vi "DEMO_08_PID_Use.vi"() -> ()   [LabVIEW 2014]
uses:
  <vilib>/Instr/_visa.llb/VISA Configure Serial Port (Instr).vi
panel:
  in  "停止 3":bool
  in  "停止 2":bool
  in  "停止":bool
  in  "开启 3":bool
  in  "开启 2":bool
  in  "开启":bool
  in  "读取 3":bool
  in  "读取 2":bool
  in  "读取":bool
  in  "P 3":dbl
  in  "设置 3":bool
  in  "D 3":dbl
  in  "I 3":dbl
  in  "P 2":dbl
  in  "设置 2":bool
  in  "D 2":dbl
  in  "I 2":dbl
  in  "P":dbl
  in  "设置":bool
  in  "D":dbl
  in  "I":dbl
  in  "打开串口":bool
  in  "上位机控制":bool
  in  "波特率":u32(ring)=9600 items=["75"=75, "110"=110, "134"=134, "150"=150, "300"=300, "600"=600, "1200"=1200, "1800"=1800, "2400"=2400, "4800"=4800, "7200"=7200, "9600"=9600, "14400"=14400, "19200"=19200, "28800"=28800, "38400"=38400, "56000"=56000, "57600"=57600, "115200"=115200, "128000"=128000, "230400"=230400]
  in  "奇偶":enum16{"None", "Odd", "Even", "Mark", "Space"}(ring) caption="校验"
  in  "VISA资源名称":refnum<visa-resource-name>="COM1"
  # "上位机设定下位机PID参数~"
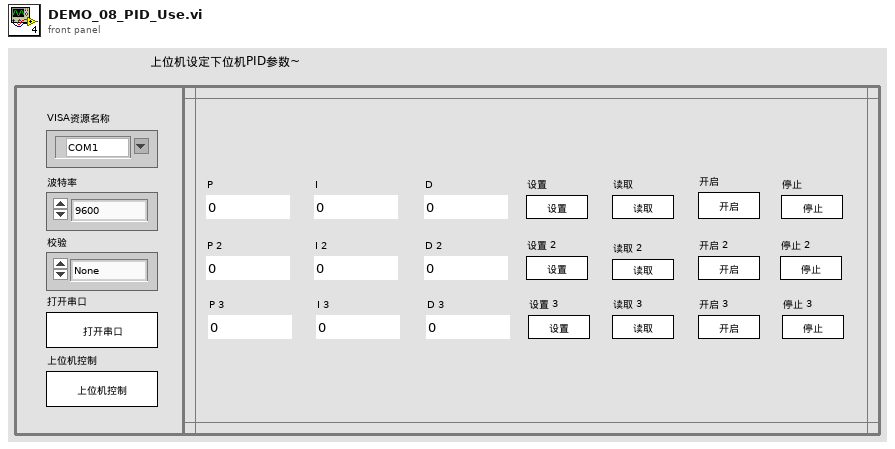
[diagram p1: front panel]
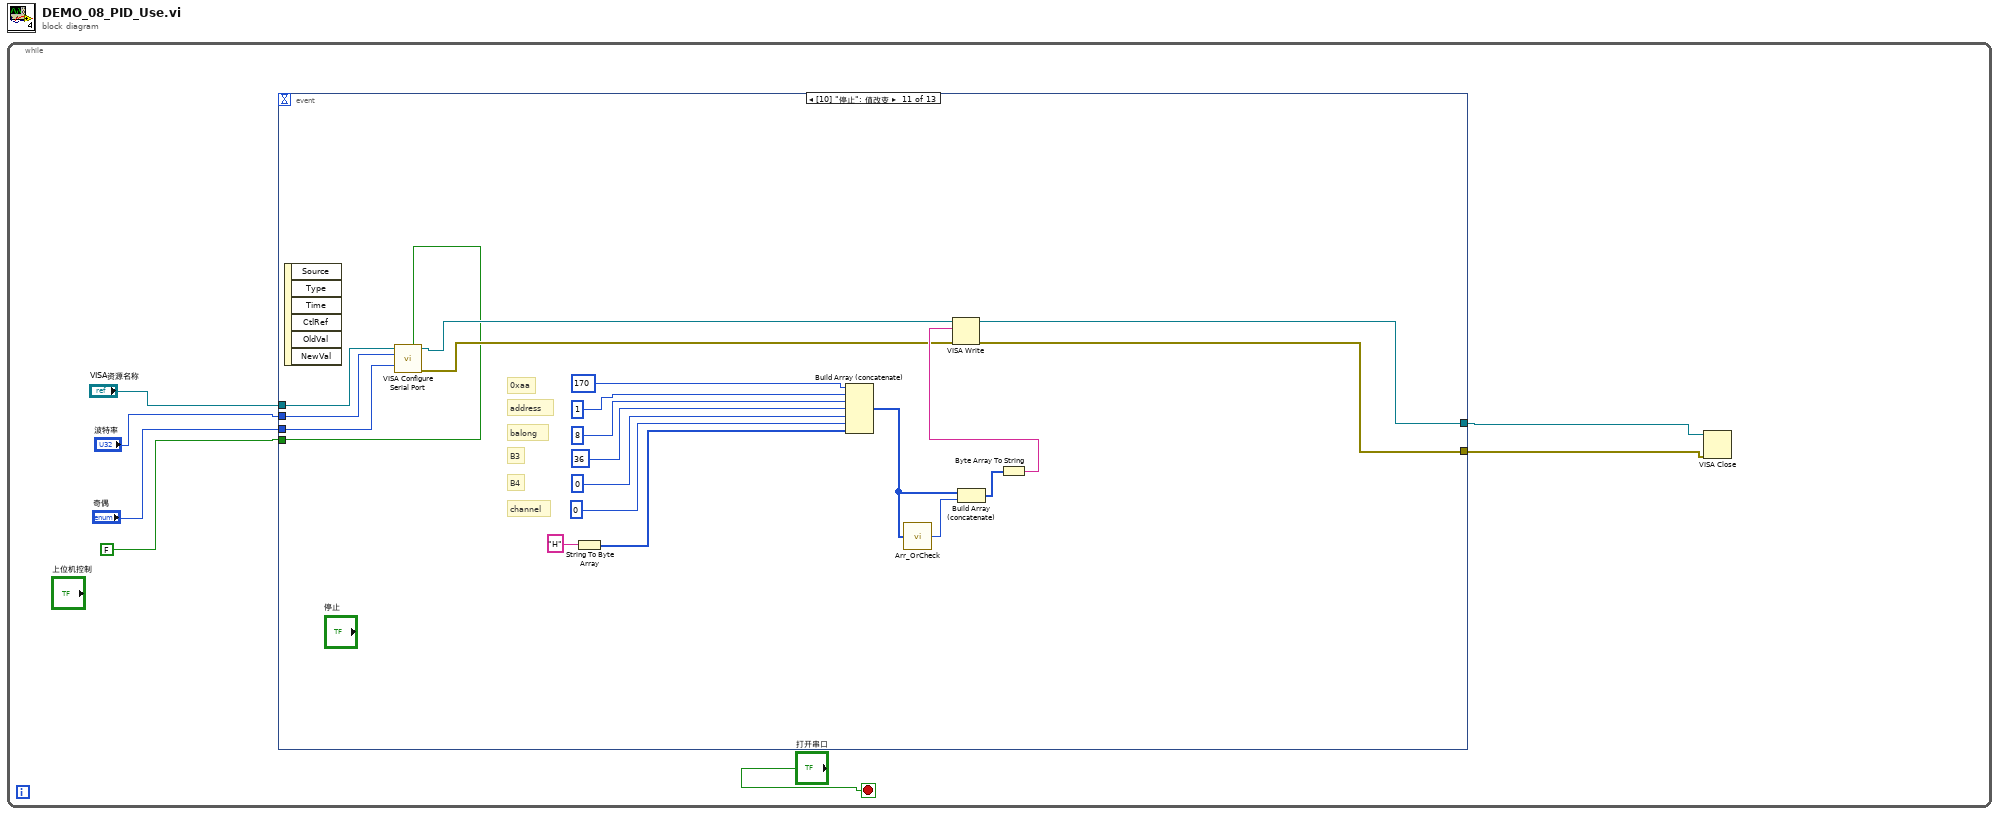
[diagram p0: block diagram]
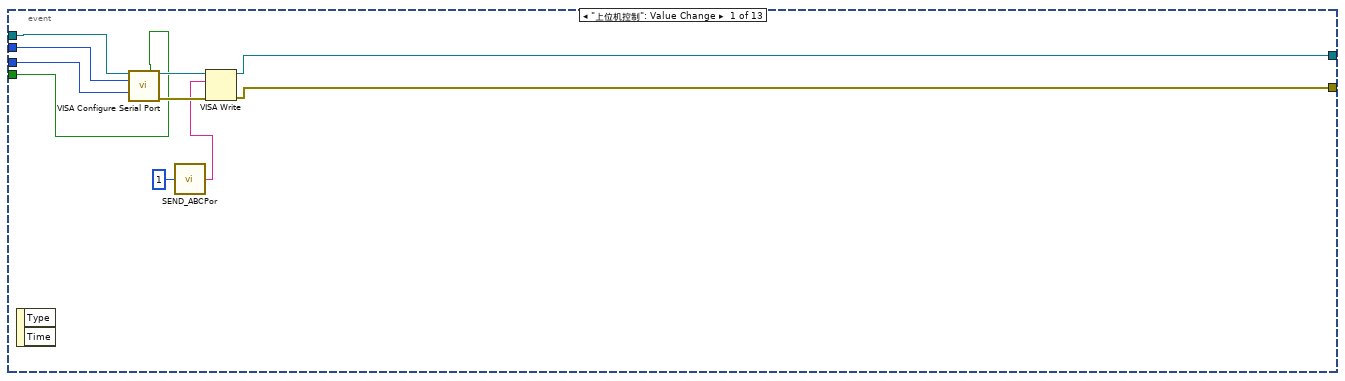
[diagram p2: hidden frame]
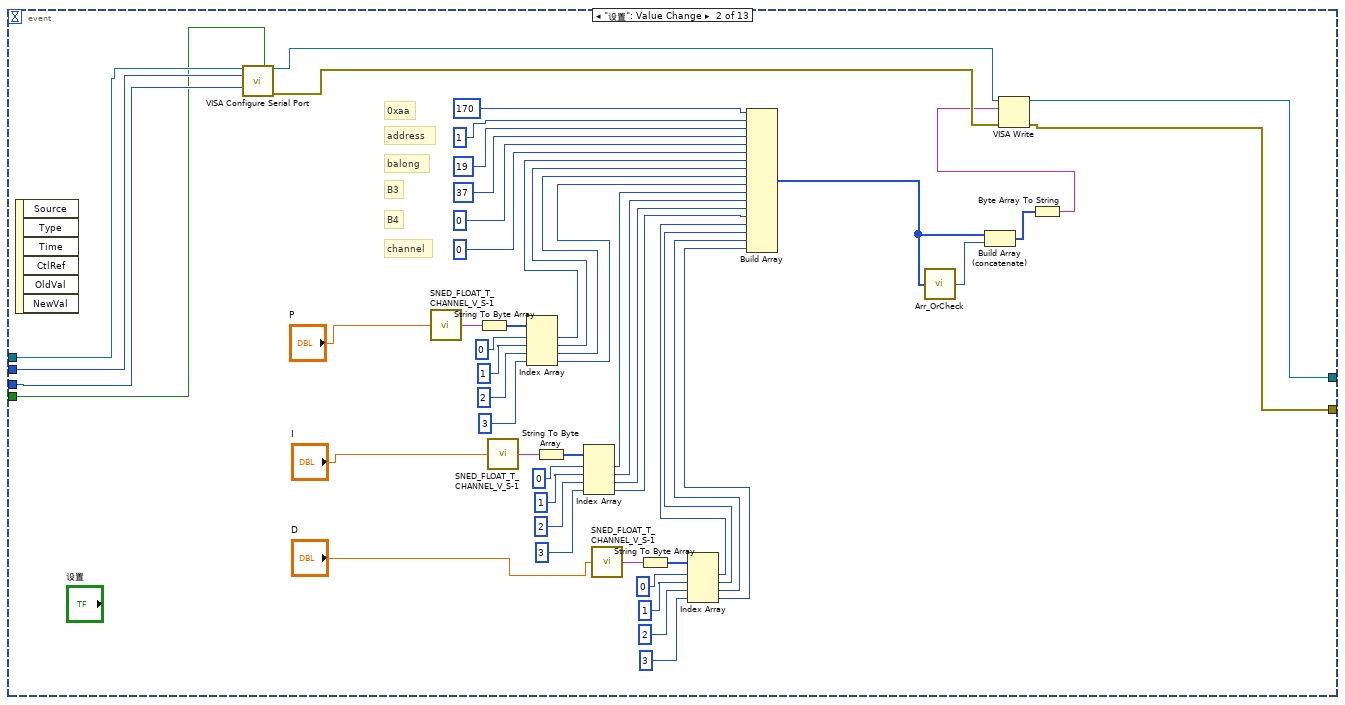
[diagram p3: hidden frame]
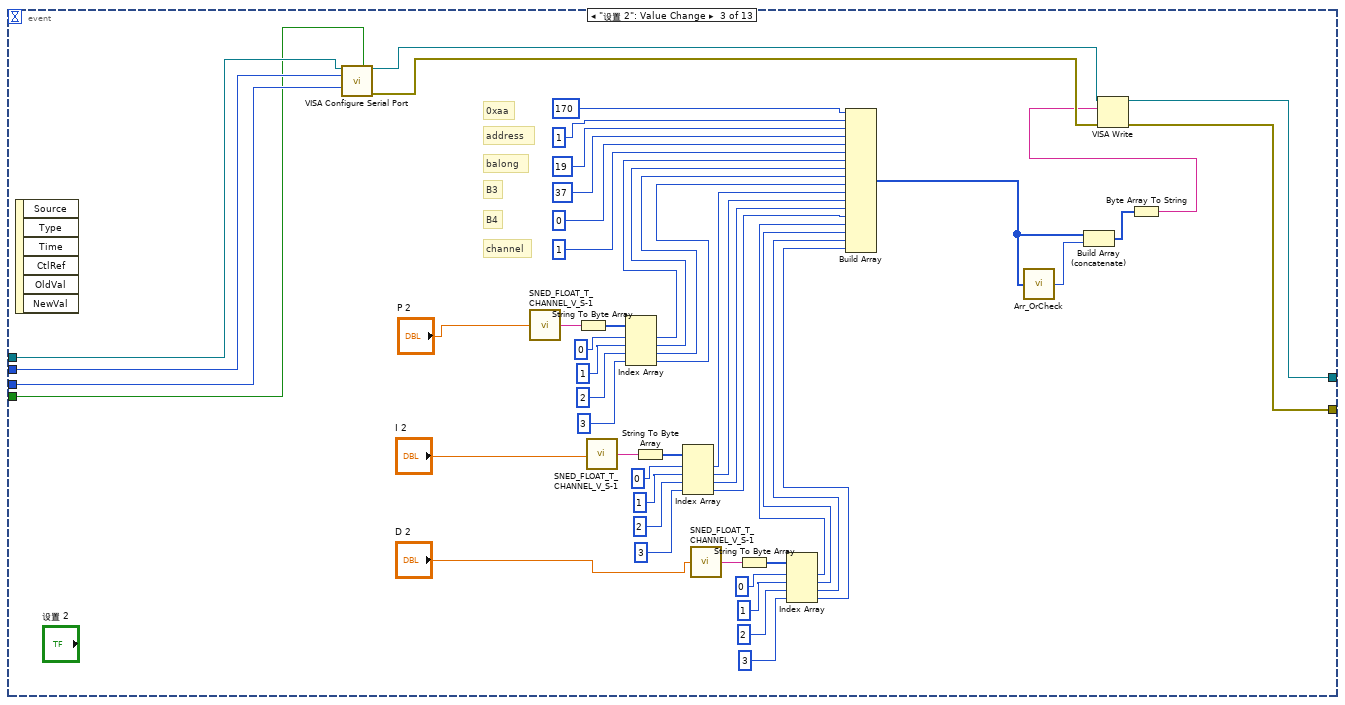
[diagram p4: hidden frame]
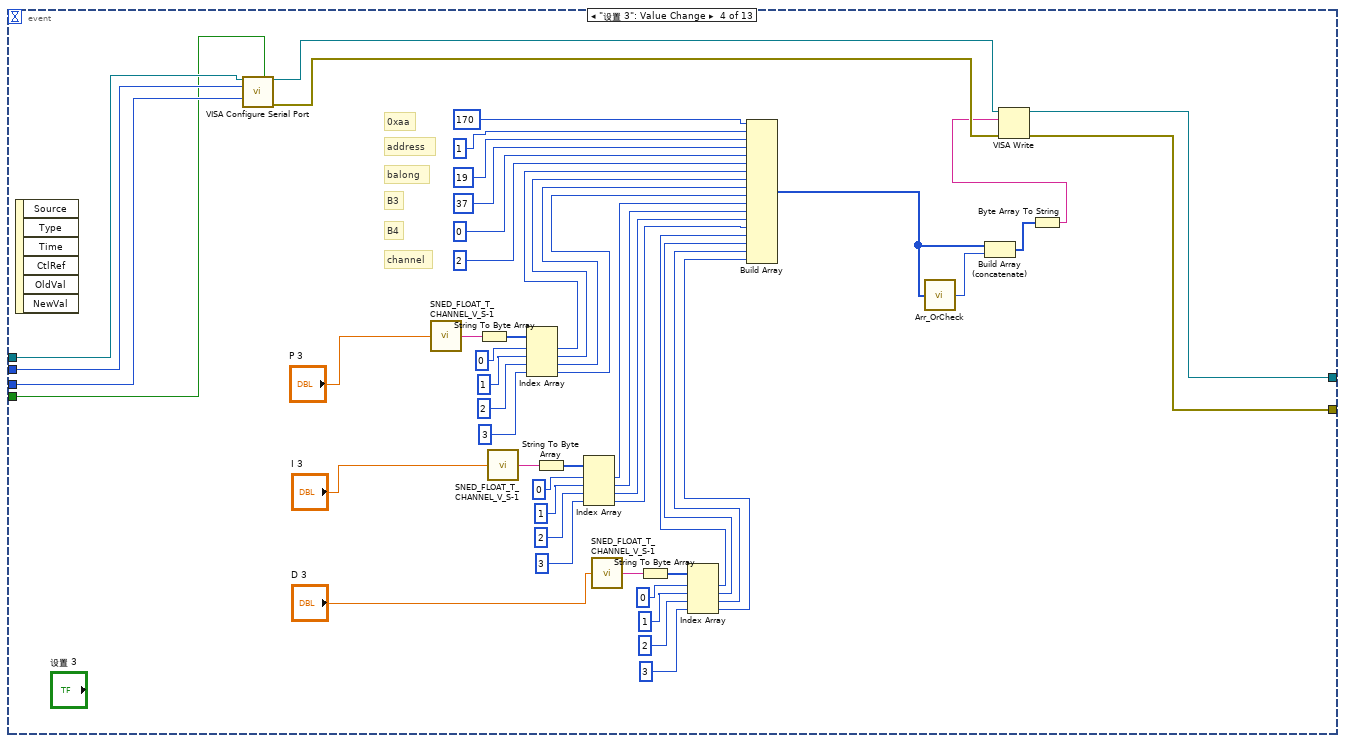
[diagram p5: hidden frame]
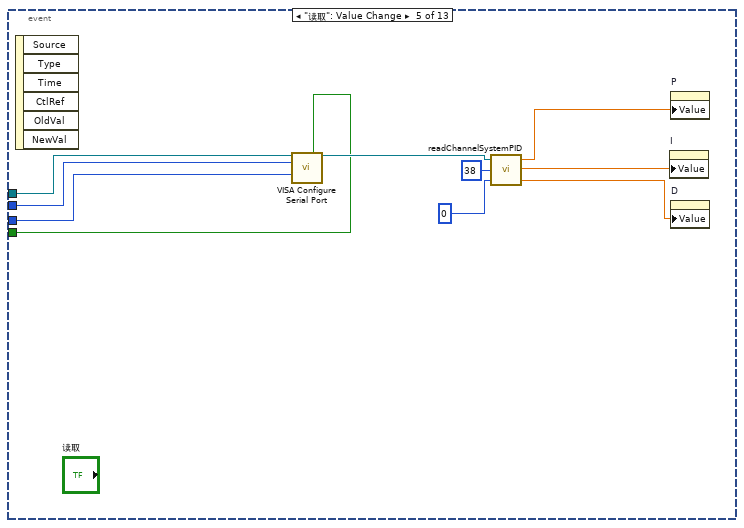
[diagram p6: hidden frame]
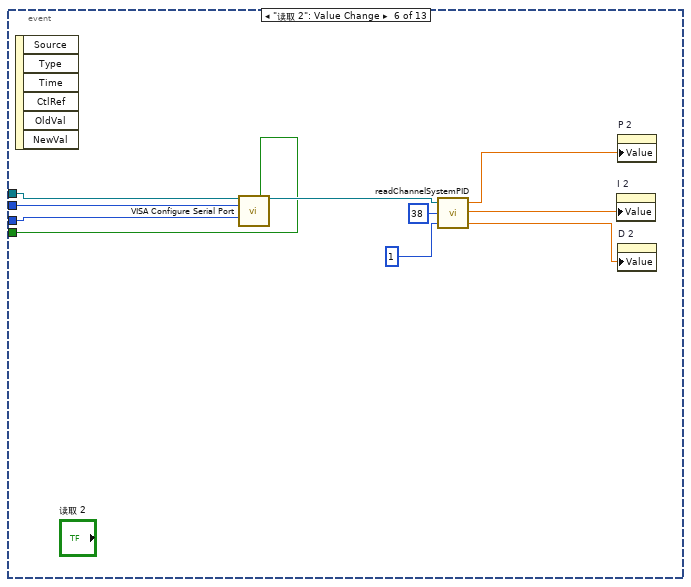
[diagram p7: hidden frame]
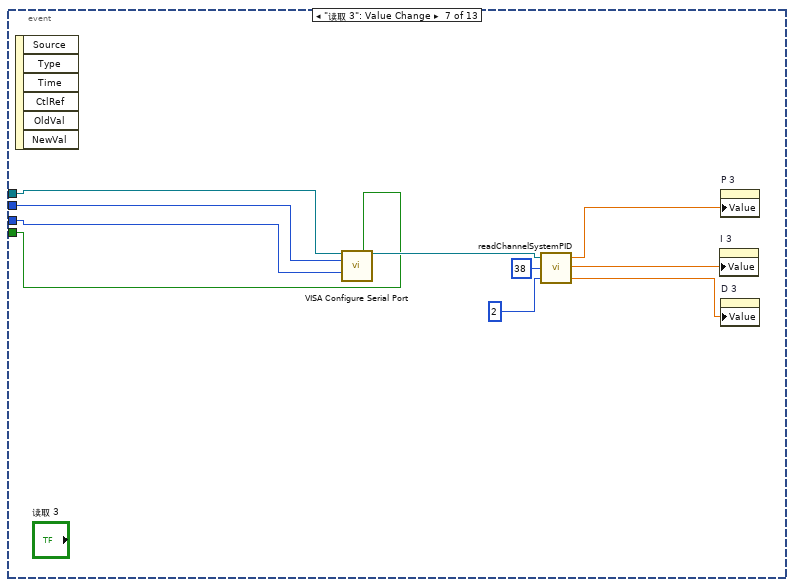
[diagram p8: hidden frame]
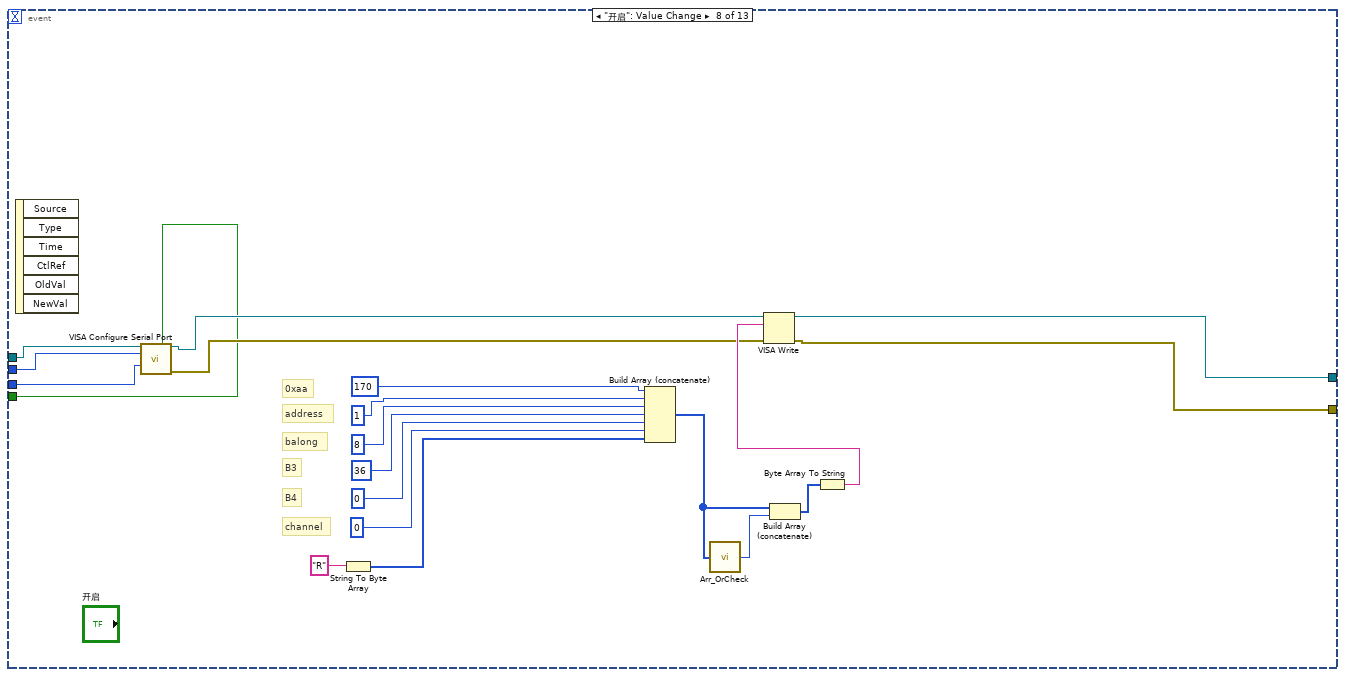
[diagram p9: hidden frame]
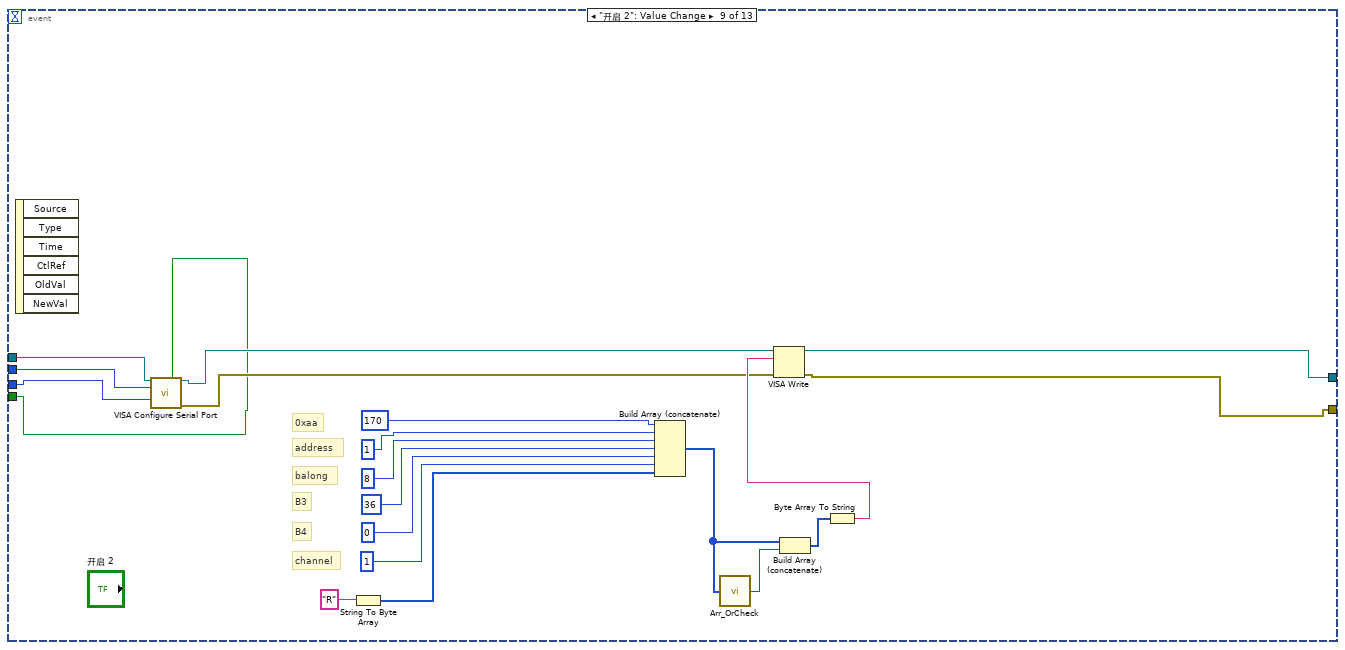
[diagram p10: hidden frame]
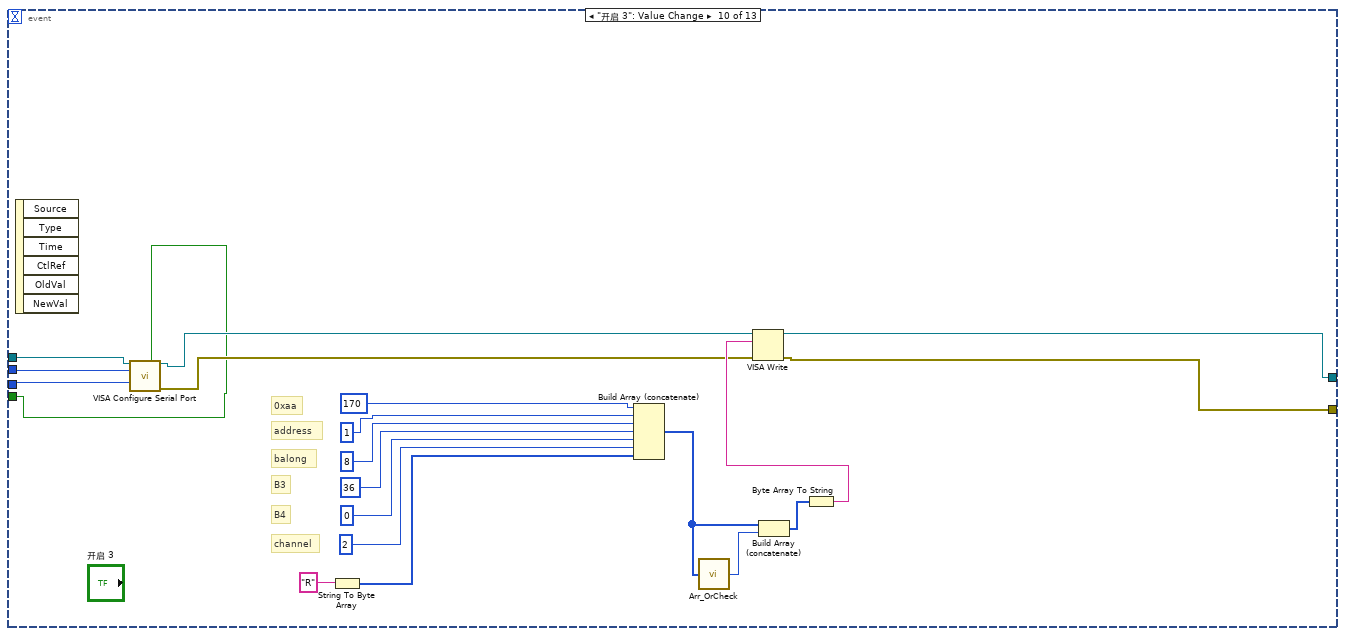
[diagram p11: hidden frame]
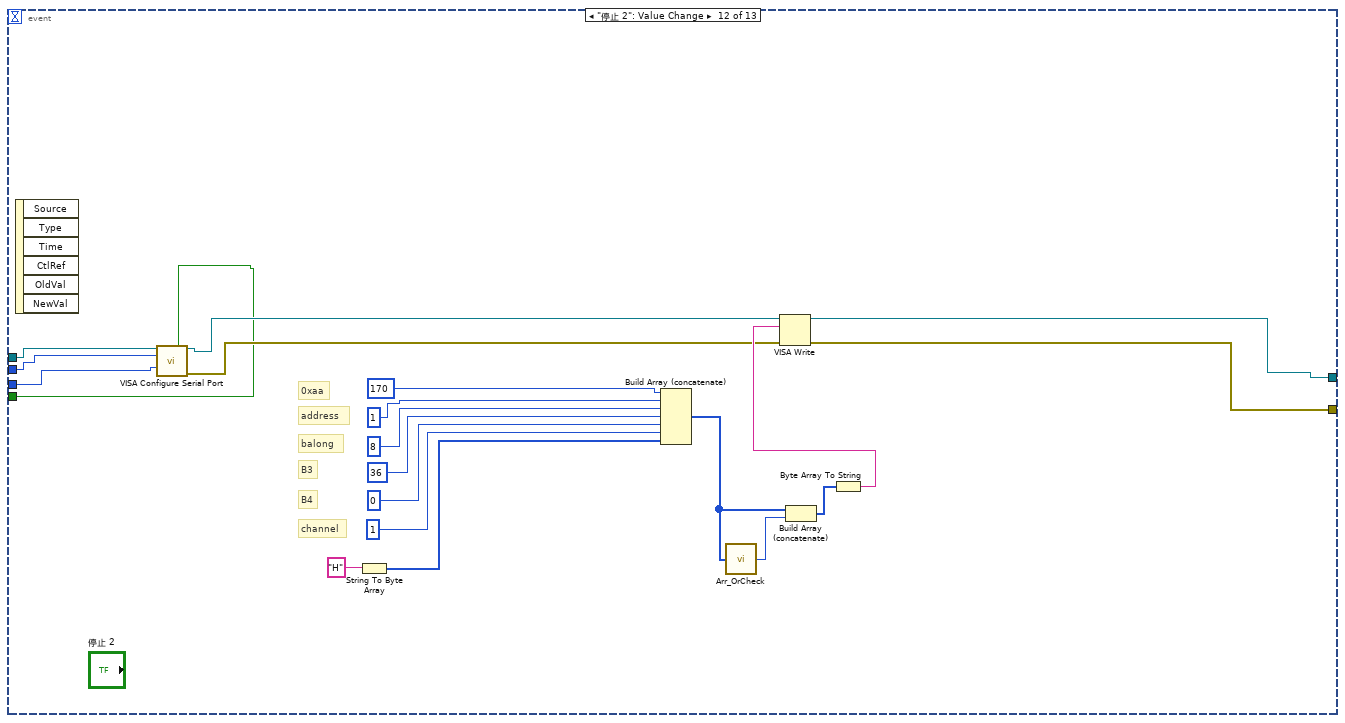
[diagram p12: hidden frame]
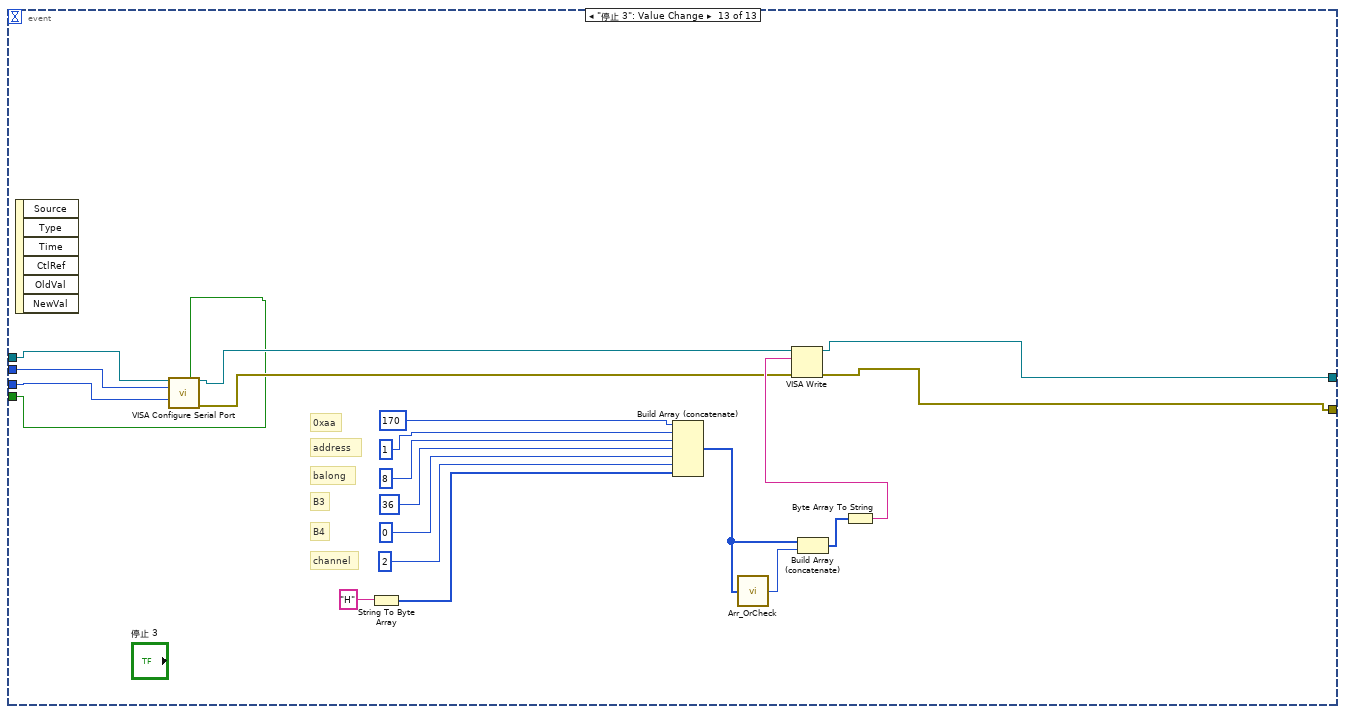
[diagram p13: hidden frame]
diagram:
  n1 = while {
    stop <- "打开串口" stop-if-true
    n2 = event shown="[10] \"停止\": 值改变" {
      selector: _ -> [_ _ _ _ _ _ _ _ _ _ _ _ _]
      dyn-events: _ -> [_ _ _ _ _ _ _ _ _ _ _ _ _]
      timeout: _ -> [_ _ _ _ _ _ _ _ _ _ _ _ _]
      tunnel: [w17 w19 w74 w121 _ _ _ w201 w226 w242 w262 w286 w302] -> w2
      tunnel: FALSE -> [w11 w23 w77 w129 w174 w181 w191 w203 w221 w243 w264 w281 w303]
      tunnel: "VISA资源名称" -> [w14 w26 w80 w132 w177 w184 w194 w206 w224 w246 w267 w284 w306]
      tunnel: "波特率" -> [w13 w25 w79 w131 w176 w183 w193 w205 w223 w245 w266 w283 w305]
      tunnel: "奇偶" -> [w12 w24 w78 w130 w175 w182 w192 w204 w222 w244 w265 w282 w304]
      tunnel: [w8 w20 w73 w122 _ _ _ w202 w225 w241 w263 w285 w301] -> w1
      event "上位机控制": Value Change {
        n3 = event-data() -> ()  [unwired: 1 in, 2 out]
        n4 = call-poly "VISA Configure Serial Port"("VISA resource name"=w14, "Enable Termination\nChar (T)"=w11, "baud rate (9600)"=w13, "parity (0:none)"=w12) -> ("VISA resource name out"=w16:refnum<visa-resource-name>, "error out"=w15:errorcluster)  [unwired: 10 in]
        n5 = call "SEND_ABCPor.vi"("设备地址 1 开始"=1) -> ("输出字符串"=w9:string)
        n6 = VISA Write(VISA resource name=w16, write buffer=w9, error in (no error)=w15) -> (VISA resource name out=w8:refnum<visa-resource-name>, error out=w17:errorcluster)  [unwired: 1 out]
      }
      event "设置": Value Change {
        # "channel"
        # "B4"
        # "B3"
        # "balong"
        # "address"
        # "0xaa"
        n7 = event-data() -> ()  [unwired: 1 in, 6 out]
        n8 = call-poly "VISA Configure Serial Port"("VISA resource name"=w26, "Enable Termination\nChar (T)"=w23, "baud rate (9600)"=w25, "parity (0:none)"=w24) -> ("VISA resource name out"=w22:refnum<visa-resource-name>, "error out"=w21:errorcluster)  [unwired: 10 in]
        n9 = call "SNED_FLOAT_T_CHANNEL_V_S-1.vi"("数据"="P") -> ("字符串"=w68:string)
        n10 = String To Byte Array(string=w68) -> (unsigned byte array=w67:u8[])
        n11 = call "SNED_FLOAT_T_CHANNEL_V_S-1.vi"("数据"="I") -> ("字符串"=w60:string)
        n12 = Index Array(array=w67, index #1=0, index #2=1, index #3=2, index #4=3) -> (element #1=w44:u8, element #2=w43:u8, element #3=w42:u8, element #4=w41:u8)
        n13 = String To Byte Array(string=w60) -> (unsigned byte array=w59:u8[])
        n14 = Index Array(array=w59, index #1=0, index #2=1, index #3=2, index #4=3) -> (element #1=w38:u8, element #2=w37:u8, element #3=w36:u8, element #4=w35:u8)
        n15 = call "SNED_FLOAT_T_CHANNEL_V_S-1.vi"("数据"="D") -> ("字符串"=w54:string)
        n16 = String To Byte Array(string=w54) -> (unsigned byte array=w53:u8[])
        n17 = Index Array(array=w53, index #1=0, index #2=1, index #3=2, index #4=3) -> (element #1=w34:u8, element #2=w33:u8, element #3=w32:u8, element #4=w31:u8)
        n18 = Build Array(170, 1, 19, 37, 0, 0, w44, w43, w42, w41, w38, w37, w36, w35, w34, w33, w32, w31) -> (w30:i32[])
        n19 = call "Arr_OrCheck.vi"("数组"=w30) -> ("抑或的数据值"=w62:u8)
        n20 = Build Array (concatenate)(w30, w62) -> (w61:i32[])
        n21 = Byte Array To String(unsigned byte array=w61) -> (string=w18:string)
        n22 = VISA Write(VISA resource name=w22, write buffer=w18, error in (no error)=w21) -> (VISA resource name out=w20:refnum<visa-resource-name>, error out=w19:errorcluster)  [unwired: 1 out]
      }
      event "设置 2": Value Change {
        # "channel"
        # "B4"
        # "B3"
        # "balong"
        # "address"
        # "0xaa"
        n23 = event-data() -> ()  [unwired: 1 in, 6 out]
        n24 = call-poly "VISA Configure Serial Port"("VISA resource name"=w80, "Enable Termination\nChar (T)"=w77, "baud rate (9600)"=w79, "parity (0:none)"=w78) -> ("VISA resource name out"=w76:refnum<visa-resource-name>, "error out"=w75:errorcluster)  [unwired: 10 in]
        n25 = call "SNED_FLOAT_T_CHANNEL_V_S-1.vi"("数据"="P 2") -> ("字符串"=w119:string)
        n26 = String To Byte Array(string=w119) -> (unsigned byte array=w118:u8[])
        n27 = call "SNED_FLOAT_T_CHANNEL_V_S-1.vi"("数据"="I 2") -> ("字符串"=w111:string)
        n28 = Index Array(array=w118, index #1=0, index #2=1, index #3=2, index #4=3) -> (element #1=w95:u8, element #2=w94:u8, element #3=w93:u8, element #4=w92:u8)
        n29 = String To Byte Array(string=w111) -> (unsigned byte array=w110:u8[])
        n30 = Index Array(array=w110, index #1=0, index #2=1, index #3=2, index #4=3) -> (element #1=w89:u8, element #2=w88:u8, element #3=w87:u8, element #4=w86:u8)
        n31 = call "SNED_FLOAT_T_CHANNEL_V_S-1.vi"("数据"="D 2") -> ("字符串"=w105:string)
        n32 = String To Byte Array(string=w105) -> (unsigned byte array=w104:u8[])
        n33 = Index Array(array=w104, index #1=0, index #2=1, index #3=2, index #4=3) -> (element #1=w85:u8, element #2=w84:u8, element #3=w83:u8, element #4=w82:u8)
        n34 = Build Array(170, 1, 19, 37, 0, 1, w95, w94, w93, w92, w89, w88, w87, w86, w85, w84, w83, w82) -> (w81:i32[])
        n35 = call "Arr_OrCheck.vi"("数组"=w81) -> ("抑或的数据值"=w113:u8)
        n36 = Build Array (concatenate)(w81, w113) -> (w112:i32[])
        n37 = Byte Array To String(unsigned byte array=w112) -> (string=w72:string)
        n38 = VISA Write(VISA resource name=w76, write buffer=w72, error in (no error)=w75) -> (VISA resource name out=w73:refnum<visa-resource-name>, error out=w74:errorcluster)  [unwired: 1 out]
      }
      event "设置 3": Value Change {
        # "channel"
        # "B4"
        # "B3"
        # "balong"
        # "address"
        # "0xaa"
        n39 = event-data() -> ()  [unwired: 1 in, 6 out]
        n40 = call-poly "VISA Configure Serial Port"("VISA resource name"=w132, "Enable Termination\nChar (T)"=w129, "baud rate (9600)"=w131, "parity (0:none)"=w130) -> ("VISA resource name out"=w128:refnum<visa-resource-name>, "error out"=w127:errorcluster)  [unwired: 10 in]
        n41 = call "SNED_FLOAT_T_CHANNEL_V_S-1.vi"("数据"="P 3") -> ("字符串"=w170:string)
        n42 = String To Byte Array(string=w170) -> (unsigned byte array=w169:u8[])
        n43 = call "SNED_FLOAT_T_CHANNEL_V_S-1.vi"("数据"="I 3") -> ("字符串"=w162:string)
        n44 = Index Array(array=w169, index #1=0, index #2=1, index #3=2, index #4=3) -> (element #1=w146:u8, element #2=w145:u8, element #3=w144:u8, element #4=w120:u8)
        n45 = String To Byte Array(string=w162) -> (unsigned byte array=w161:u8[])
        n46 = Index Array(array=w161, index #1=0, index #2=1, index #3=2, index #4=3) -> (element #1=w141:u8, element #2=w140:u8, element #3=w139:u8, element #4=w138:u8)
        n47 = call "SNED_FLOAT_T_CHANNEL_V_S-1.vi"("数据"="D 3") -> ("字符串"=w156:string)
        n48 = String To Byte Array(string=w156) -> (unsigned byte array=w155:u8[])
        n49 = Index Array(array=w155, index #1=0, index #2=1, index #3=2, index #4=3) -> (element #1=w137:u8, element #2=w136:u8, element #3=w135:u8, element #4=w134:u8)
        n50 = Build Array(170, 1, 19, 37, 0, 2, w146, w145, w144, w120, w141, w140, w139, w138, w137, w136, w135, w134) -> (w133:i32[])
        n51 = call "Arr_OrCheck.vi"("数组"=w133) -> ("抑或的数据值"=w164:u8)
        n52 = Build Array (concatenate)(w133, w164) -> (w163:i32[])
        n53 = Byte Array To String(unsigned byte array=w163) -> (string=w123:string)
        n54 = VISA Write(VISA resource name=w128, write buffer=w123, error in (no error)=w127) -> (VISA resource name out=w122:refnum<visa-resource-name>, error out=w121:errorcluster)  [unwired: 1 out]
      }
      event "读取": Value Change {
        n55 = event-data() -> ()  [unwired: 1 in, 6 out]
        n56 = call-poly "VISA Configure Serial Port"("VISA resource name"=w177, "Enable Termination\nChar (T)"=w174, "baud rate (9600)"=w176, "parity (0:none)"=w175) -> ("VISA resource name out"=w178:refnum<visa-resource-name>)  [unwired: 10 in, 1 out]
        n57 = call "readChannelSystemPID.vi"("通道号"=0, "B3"=38, "VISA resource name out 2"=w178) -> ("D"=w171:dbl, "I"=w172:dbl, "P"=w173:dbl)
        n58 = property on="I" class="DigNum (严格)"("Value"=w172) -> ()  [unwired: 2 in, 2 out]
        n59 = property on="P" class="DigNum (严格)"("Value"=w173) -> ()  [unwired: 2 in, 2 out]
        n60 = property on="D" class="DigNum (严格)"("Value"=w171) -> ()  [unwired: 2 in, 2 out]
      }
      event "读取 2": Value Change {
        n61 = event-data() -> ()  [unwired: 1 in, 6 out]
        n62 = call-poly "VISA Configure Serial Port"("VISA resource name"=w184, "Enable Termination\nChar (T)"=w181, "baud rate (9600)"=w183, "parity (0:none)"=w182) -> ("VISA resource name out"=w188:refnum<visa-resource-name>)  [unwired: 10 in, 1 out]
        n63 = call "readChannelSystemPID.vi"("通道号"=1, "B3"=38, "VISA resource name out 2"=w188) -> ("D"=w185:dbl, "I"=w186:dbl, "P"=w187:dbl)
        n64 = property on="I 2" class="DigNum (严格)"("Value"=w186) -> ()  [unwired: 2 in, 2 out]
        n65 = property on="P 2" class="DigNum (严格)"("Value"=w187) -> ()  [unwired: 2 in, 2 out]
        n66 = property on="D 2" class="DigNum (严格)"("Value"=w185) -> ()  [unwired: 2 in, 2 out]
      }
      event "读取 3": Value Change {
        n67 = event-data() -> ()  [unwired: 1 in, 6 out]
        n68 = call-poly "VISA Configure Serial Port"("VISA resource name"=w194, "Enable Termination\nChar (T)"=w191, "baud rate (9600)"=w193, "parity (0:none)"=w192) -> ("VISA resource name out"=w198:refnum<visa-resource-name>)  [unwired: 10 in, 1 out]
        n69 = call "readChannelSystemPID.vi"("通道号"=2, "B3"=38, "VISA resource name out 2"=w198) -> ("D"=w195:dbl, "I"=w196:dbl, "P"=w197:dbl)
        n70 = property on="I 3" class="DigNum (严格)"("Value"=w196) -> ()  [unwired: 2 in, 2 out]
        n71 = property on="P 3" class="DigNum (严格)"("Value"=w197) -> ()  [unwired: 2 in, 2 out]
        n72 = property on="D 3" class="DigNum (严格)"("Value"=w195) -> ()  [unwired: 2 in, 2 out]
      }
      event "开启": Value Change {
        # "channel"
        # "B4"
        # "B3"
        # "balong"
        # "address"
        # "0xaa"
        n73 = event-data() -> ()  [unwired: 1 in, 6 out]
        n74 = call-poly "VISA Configure Serial Port"("VISA resource name"=w206, "Enable Termination\nChar (T)"=w203, "baud rate (9600)"=w205, "parity (0:none)"=w204) -> ("VISA resource name out"=w208:refnum<visa-resource-name>, "error out"=w207:errorcluster)  [unwired: 10 in]
        n75 = String To Byte Array(string="R") -> (unsigned byte array=w213:u8[])
        n76 = Build Array (concatenate)(170, 1, 8, 36, 0, 0, w213) -> (w210:i32[])
        n77 = call "Arr_OrCheck.vi"("数组"=w210) -> ("抑或的数据值"=w212:u8)
        n78 = Build Array (concatenate)(w210, w212) -> (w211:i32[])
        n79 = Byte Array To String(unsigned byte array=w211) -> (string=w209:string)
        n80 = VISA Write(VISA resource name=w208, write buffer=w209, error in (no error)=w207) -> (VISA resource name out=w202:refnum<visa-resource-name>, error out=w201:errorcluster)  [unwired: 1 out]
      }
      event "开启 2": Value Change {
        # "channel"
        # "B4"
        # "B3"
        # "balong"
        # "address"
        # "0xaa"
        n81 = event-data() -> ()  [unwired: 1 in, 6 out]
        n82 = call-poly "VISA Configure Serial Port"("VISA resource name"=w224, "Enable Termination\nChar (T)"=w221, "baud rate (9600)"=w223, "parity (0:none)"=w222) -> ("VISA resource name out"=w228:refnum<visa-resource-name>, "error out"=w227:errorcluster)  [unwired: 10 in]
        n83 = String To Byte Array(string="R") -> (unsigned byte array=w233:u8[])
        n84 = Build Array (concatenate)(170, 1, 8, 36, 0, 1, w233) -> (w230:i32[])
        n85 = call "Arr_OrCheck.vi"("数组"=w230) -> ("抑或的数据值"=w232:u8)
        n86 = Build Array (concatenate)(w230, w232) -> (w231:i32[])
        n87 = Byte Array To String(unsigned byte array=w231) -> (string=w229:string)
        n88 = VISA Write(VISA resource name=w228, write buffer=w229, error in (no error)=w227) -> (VISA resource name out=w225:refnum<visa-resource-name>, error out=w226:errorcluster)  [unwired: 1 out]
      }
      event "开启 3": Value Change {
        # "channel"
        # "B4"
        # "B3"
        # "balong"
        # "address"
        # "0xaa"
        n89 = event-data() -> ()  [unwired: 1 in, 6 out]
        n90 = call-poly "VISA Configure Serial Port"("VISA resource name"=w246, "Enable Termination\nChar (T)"=w243, "baud rate (9600)"=w245, "parity (0:none)"=w244) -> ("VISA resource name out"=w248:refnum<visa-resource-name>, "error out"=w247:errorcluster)  [unwired: 10 in]
        n91 = String To Byte Array(string="R") -> (unsigned byte array=w253:u8[])
        n92 = Build Array (concatenate)(170, 1, 8, 36, 0, 2, w253) -> (w250:i32[])
        n93 = call "Arr_OrCheck.vi"("数组"=w250) -> ("抑或的数据值"=w252:u8)
        n94 = Build Array (concatenate)(w250, w252) -> (w251:i32[])
        n95 = Byte Array To String(unsigned byte array=w251) -> (string=w249:string)
        n96 = VISA Write(VISA resource name=w248, write buffer=w249, error in (no error)=w247) -> (VISA resource name out=w241:refnum<visa-resource-name>, error out=w242:errorcluster)  [unwired: 1 out]
      }
      event "停止": Value Change {
        # "channel"
        # "B4"
        # "B3"
        # "balong"
        # "address"
        # "0xaa"
        n97 = event-data() -> ()  [unwired: 1 in, 6 out]
        n98 = call-poly "VISA Configure Serial Port"("VISA resource name"=w267, "Enable Termination\nChar (T)"=w264, "baud rate (9600)"=w266, "parity (0:none)"=w265) -> ("VISA resource name out"=w269:refnum<visa-resource-name>, "error out"=w268:errorcluster)  [unwired: 10 in]
        n99 = String To Byte Array(string="H") -> (unsigned byte array=w274:u8[])
        n100 = Build Array (concatenate)(170, 1, 8, 36, 0, 0, w274) -> (w271:i32[])
        n101 = call "Arr_OrCheck.vi"("数组"=w271) -> ("抑或的数据值"=w273:u8)
        n102 = Build Array (concatenate)(w271, w273) -> (w272:i32[])
        n103 = Byte Array To String(unsigned byte array=w272) -> (string=w270:string)
        n104 = VISA Write(VISA resource name=w269, write buffer=w270, error in (no error)=w268) -> (VISA resource name out=w263:refnum<visa-resource-name>, error out=w262:errorcluster)  [unwired: 1 out]
      }
      event "停止 2": Value Change {
        # "channel"
        # "B4"
        # "B3"
        # "balong"
        # "address"
        # "0xaa"
        n105 = event-data() -> ()  [unwired: 1 in, 6 out]
        n106 = call-poly "VISA Configure Serial Port"("VISA resource name"=w284, "Enable Termination\nChar (T)"=w281, "baud rate (9600)"=w283, "parity (0:none)"=w282) -> ("VISA resource name out"=w288:refnum<visa-resource-name>, "error out"=w287:errorcluster)  [unwired: 10 in]
        n107 = String To Byte Array(string="H") -> (unsigned byte array=w293:u8[])
        n108 = Build Array (concatenate)(170, 1, 8, 36, 0, 1, w293) -> (w290:i32[])
        n109 = call "Arr_OrCheck.vi"("数组"=w290) -> ("抑或的数据值"=w292:u8)
        n110 = Build Array (concatenate)(w290, w292) -> (w291:i32[])
        n111 = Byte Array To String(unsigned byte array=w291) -> (string=w289:string)
        n112 = VISA Write(VISA resource name=w288, write buffer=w289, error in (no error)=w287) -> (VISA resource name out=w285:refnum<visa-resource-name>, error out=w286:errorcluster)  [unwired: 1 out]
      }
      event "停止 3": Value Change {
        # "channel"
        # "B4"
        # "B3"
        # "balong"
        # "address"
        # "0xaa"
        n113 = event-data() -> ()  [unwired: 1 in, 6 out]
        n114 = call-poly "VISA Configure Serial Port"("VISA resource name"=w306, "Enable Termination\nChar (T)"=w303, "baud rate (9600)"=w305, "parity (0:none)"=w304) -> ("VISA resource name out"=w308:refnum<visa-resource-name>, "error out"=w307:errorcluster)  [unwired: 10 in]
        n115 = String To Byte Array(string="H") -> (unsigned byte array=w313:u8[])
        n116 = Build Array (concatenate)(170, 1, 8, 36, 0, 2, w313) -> (w310:i32[])
        n117 = call "Arr_OrCheck.vi"("数组"=w310) -> ("抑或的数据值"=w312:u8)
        n118 = Build Array (concatenate)(w310, w312) -> (w311:i32[])
        n119 = Byte Array To String(unsigned byte array=w311) -> (string=w309:string)
        n120 = VISA Write(VISA resource name=w308, write buffer=w309, error in (no error)=w307) -> (VISA resource name out=w301:refnum<visa-resource-name>, error out=w302:errorcluster)  [unwired: 1 out]
      }
    }
    n121 = VISA Close(VISA resource name=w1, error in (no error)=w2) -> ()  [unwired: 1 out]
  }
